vi "Init.vi"(8 "error in (no error)":errorcluster, 11 "Device Descriptor in":string) -> (0 "error out":errorcluster, 3 "PBP Driver":refnum<class "heater_parent.lvclass">)   [LabVIEW 2020, in "Polar Bear Plus All-in-One Plugin.lvlib"]
uses:
  Polar Bear Plus All-in-One Plugin.lvlib
  Typedefs/Init.vi States.ctl
  <instrlib>/RxnRover/Driver Polar Bear Plus/heater_flow_synthesiser/heater_flow_synthesiser.lvclass
  <instrlib>/RxnRover/Driver Polar Bear Plus/heater_explorer/heater_explorer.lvclass
  <instrlib>/RxnRover/Driver Polar Bear Plus/heater_parent/heater_parent.lvclass
  C:/Program Files (x86)/National Instruments/LabVIEW 2020/instr.lib/RxnRover/Driver Polar Bear Plus/heater_parent/heater_parent.lvclass
panel:
  in  "Device Type":string(combo)="PBP Flow Synthesiser"
  in  "IP Address":string
  in  "Connect Btn":bool
  # "1. Device Type"
  # "2. Device IP Address"
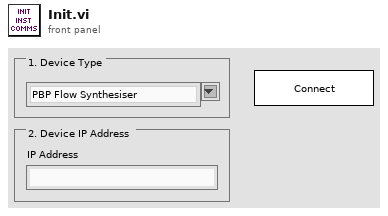
[diagram p1: front panel]
types:
  T1 = typedef "Polar Bear Plus All-in-One Plugin.lvlib/Init.vi States.ctl" = enum16{"Waiting for connection", "Connecting", "Successful connection", "Failed to connect", "Closing"}
  T2 = enum32{"Invalid", "Standard", "Closed", "Hidden", "Minimized", "Maximized"}
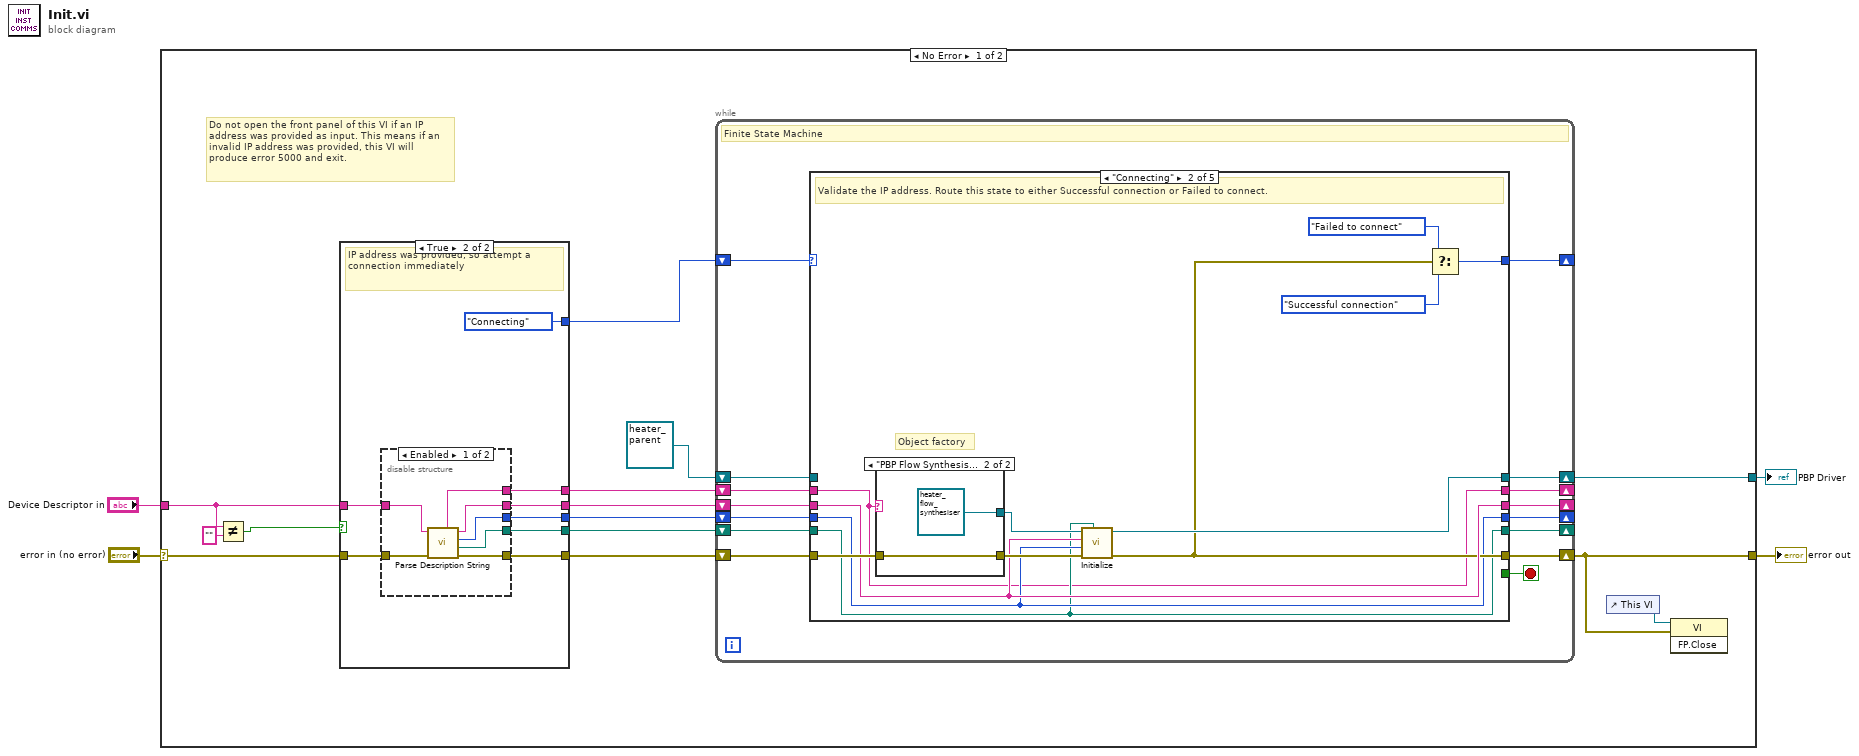
[diagram p0: block diagram]
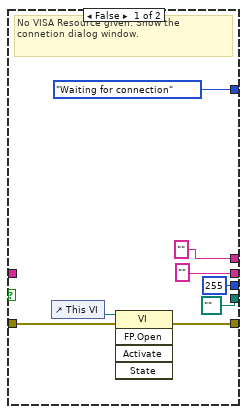
[diagram p2: hidden frame]
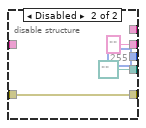
[diagram p3: hidden frame]
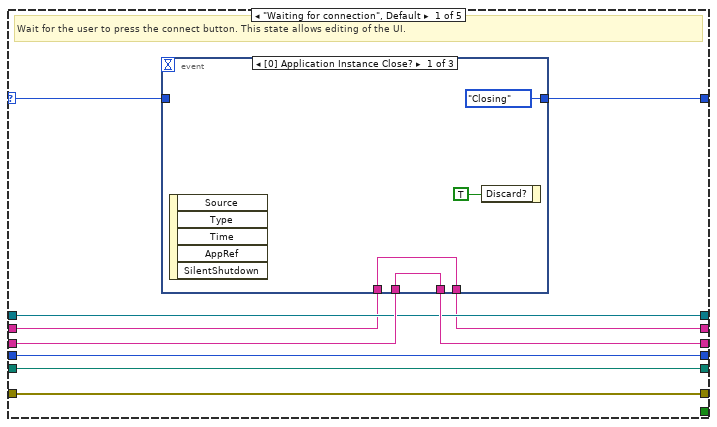
[diagram p4: hidden frame]
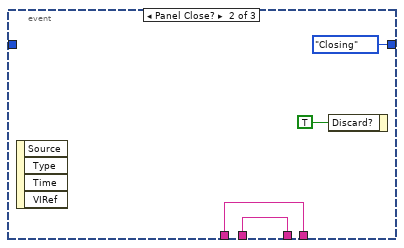
[diagram p5: hidden frame]
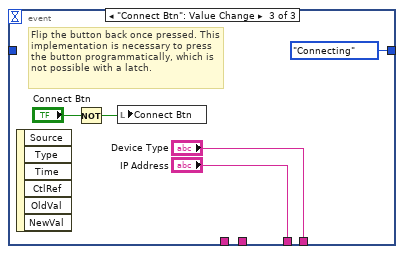
[diagram p6: hidden frame]
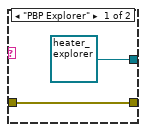
[diagram p7: hidden frame]
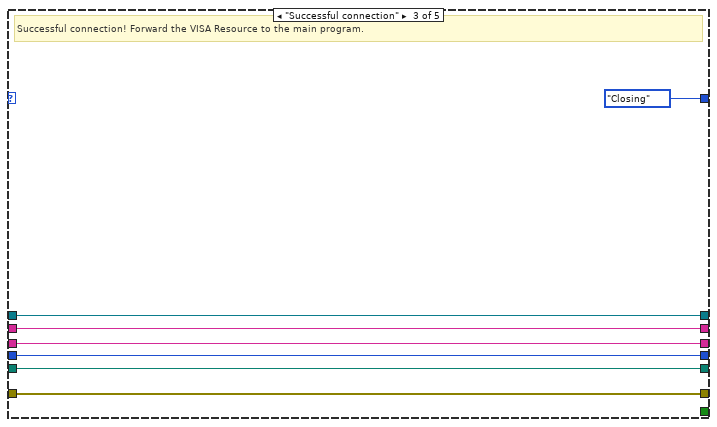
[diagram p8: hidden frame]
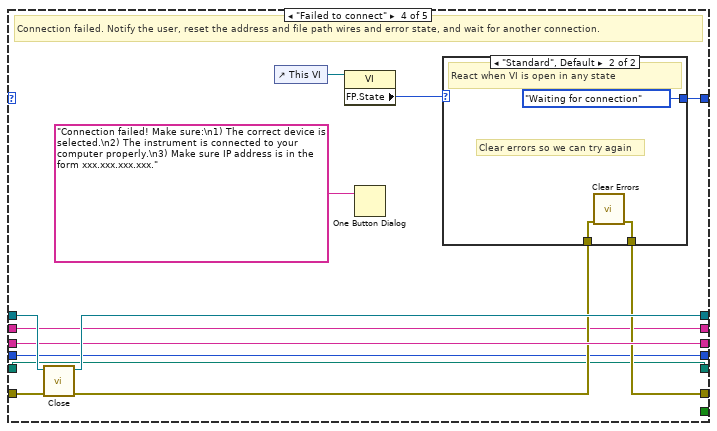
[diagram p9: hidden frame]
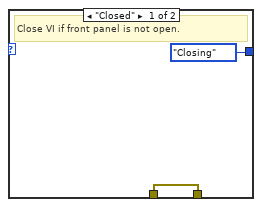
[diagram p10: hidden frame]
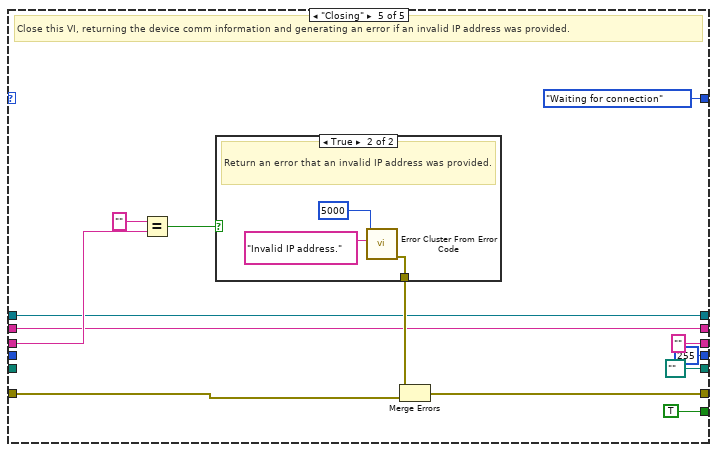
[diagram p11: hidden frame]
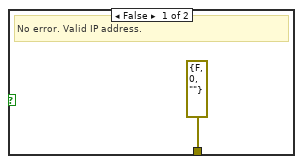
[diagram p12: hidden frame]
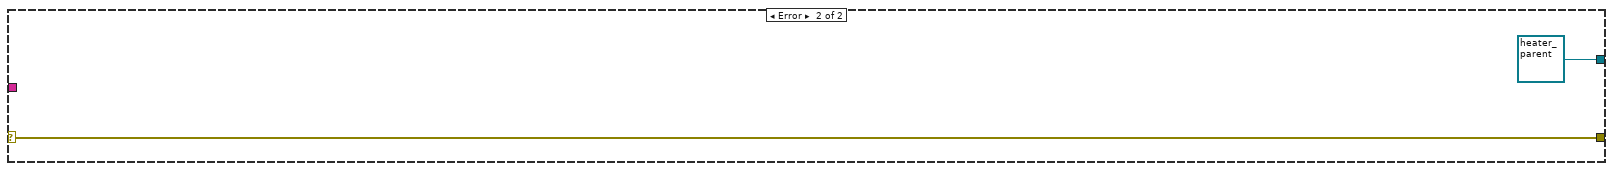
[diagram p13: hidden frame]
diagram:
  n1 = case shown="No Error" "error in (no error)" {
    selector: "error in (no error)" -> [w15 w143]
    tunnel: [w17 w143] -> w3
    tunnel: "Device Descriptor in" -> [w12 _]
    tunnel: [w10 refnum<class "heater_parent.lvclass"> refnum ("polar_bear_plus_drivers.lvlib:heater_parent.lvclass")] -> w1
    frame No Error {
      # "Do not open the front panel of this VI if an IP address was provided as input. This means if an invalid IP address was provided, this VI will produce error 5000 and exit."
      n2 = Not Equal?(x=w12, y="" ("x")) -> (x != y?=w9:bool)
      n3 = case shown="True" w9 {
        tunnel: w15 -> [w25 w34]
        tunnel: [w24 w32] -> w14
        tunnel: [Init.vi_States."Waiting for connection" Init.vi_States."Connecting"] -> w13
        tunnel: w12 -> [_ w31]
        tunnel: ["" ("READ;WRITE Files in") w30] -> w11
        tunnel: [u8 255 ("Modbus Address") w29] -> w7
        tunnel: [path "" ("Data Directory") w28] -> w6
        tunnel: ["" ("READ;WRITE Files in") w27] -> w5
        frame False {
          # "No VISA Resource given. Show the connetion dialog window."
          n4 = control-ref of="This VI"() -> (w26:refnum<vi>)
          n5 = invoke class="VI" method="FP.Open"(reference=w26, error in=w25) -> (error out=w24:errorcluster)  [unwired: 3 in, 4 out]
        }
        frame True {
          # "IP address was provided, so attempt a connection immediately"
          n6 = disable-structure shown="Enabled" {
            disable-tunnel: w34 -> [w41 w42]
            disable-tunnel: [w40 w42] -> w32
            disable-tunnel: w31 -> [w39 _]
            disable-tunnel: [w38 "" ("IP Address")] -> w30
            disable-tunnel: [w37 u8 255 ("Modbus Address")] -> w29
            disable-tunnel: [w36 path "" ("Data Directory")] -> w28
            disable-tunnel: [w35 _] -> w27
            frame Enabled {
              n7 = call <instrlib>:"Parse Description String.vi"("error in (no error)"=w41, "Description String"=w39) -> ("error out"=w40:errorcluster, "Data Directory"=w36:path, "Modbus Address"=w37:u8, "IP Address"=w38:string, "Device Type"=w35:string)  [unwired: 5 in]
            }
            frame Disabled {
            }
          }
        }
      }
      n8 = while {
        shift-right: [w59] -> _
        shift-left: w13 -> [w60]
        shift-right: [w52] -> _
        shift-left: w11 -> [w57]
        shift-right: [w55] -> w17
        shift-left: w14 -> [w56]
        shift-right: [w54] -> w10
        shift-left: refnum<class "heater_parent.lvclass"> refnum ("polar_bear_plus_drivers.lvlib:heater_parent.lvclass") -> [w53]
        shift-right: [w49] -> _
        shift-left: w7 -> [w51]
        shift-right: [w48] -> _
        shift-left: w6 -> [w50]
        shift-right: [w47] -> _
        shift-left: w5 -> [w46]
        stop <- w58 stop-if-true
        # "Finite State Machine"
        n9 = case shown="\"Connecting\"" w60 {
          selector: w60 -> [w70 _ _ _ _]
          tunnel: [w69 w95 Init.vi_States."Closing" w119 Init.vi_States."Waiting for connection"] -> w59
          tunnel: [_ _ _ _ TRUE] -> w58
          tunnel: [w65 w89 w104 w113 w131] -> w54
          tunnel: w57 -> [w67 w88 w103 w112 w135]
          tunnel: w56 -> [w68 w92 w105 w115 w132]
          tunnel: [w68 w87 w105 w110 w133] -> w55
          tunnel: w53 -> [w65 _ w104 w114 w131]
          tunnel: [w66 w88 w103 w112 "" ("READ;WRITE Files in")] -> w52
          tunnel: w51 -> [w64 w86 w102 w109 _]
          tunnel: w50 -> [w63 w85 w101 w108 _]
          tunnel: [w64 w86 w102 w109 u8 255 ("Modbus Address")] -> w49
          tunnel: [w63 w85 w101 w108 path "" ("Data Directory")] -> w48
          tunnel: [w62 w84 w100 w107 w125] -> w47
          tunnel: w46 -> [w61 w84 w100 w107 w125]
          frame "Waiting for connection", Default {
            # "Wait for the user to press the connect button. This state allows editing of the UI."
            n10 = event shown="[0] Application Instance Close?" {
              selector: _ -> [_ _ _]
              dyn-events: _ -> [_ _ _]
              timeout: _ -> [_ _ _]
              tunnel: [Init.vi_States."Closing" Init.vi_States."Closing" Init.vi_States."Connecting"] -> w69
              tunnel: w70 -> [_ _ _]
              tunnel: w67 -> [w72 w76 _]
              tunnel: [w72 w76 "IP Address"] -> w66
              tunnel: [w71 w75 "Device Type"] -> w62
              tunnel: w61 -> [w71 w75 _]
              event Application Instance Close? {
                n11 = event-data() -> ()  [unwired: 1 in, 5 out]
                n12 = event-data("Discard?"=TRUE) -> ()  [unwired: 1 in, 1 out]
              }
              event Panel Close? {
                n13 = event-data() -> ()  [unwired: 1 in, 4 out]
                n14 = event-data("Discard?"=TRUE) -> ()  [unwired: 1 in, 1 out]
              }
              event "Connect Btn": Value Change {
                # "Flip the button back once pressed. This implementation is necessary to press the button programmatically, which is not possible with a latch."
                n15 = event-data() -> ()  [unwired: 1 in, 6 out]
                n16 = Not(x="Connect Btn") -> (.not. x?=w81:bool)
                n17 = local write "Connect Btn"(w81) -> ()
              }
            }
          }
          frame "Connecting" {
            # "Object factory"
            # "Validate the IP address. Route this state to either Successful connection or Failed to connect."
            n18 = case shown="\"PBP Flow Synthesiser\", Default" w84 {
              tunnel: w92 -> [w97 w99]
              tunnel: [w97 w99] -> w91
              tunnel: [refnum<class "heater_explorer.lvclass"> refnum ("polar_bear_plus_drivers.lvlib:heater_explorer.lvclass") refnum<class "heater_flow_synthesiser.lvclass"> refnum ("polar_bear_plus_drivers.lvlib:heater_flow_synthesiser.lvclass")] -> w90
              frame "PBP Explorer" {
              }
              frame "PBP Flow Synthesiser", Default {
              }
            }
            n19 = call-dynamic "Initialize.vi"("start path"=w85, "error in (no error)"=w91, "Modbus Address"=w86, "IP Address"=w88, "vici_flow_actuator_parent in"=w90) -> ("error out"=w87:errorcluster, "vici_flow_actuator_parent out"=w89:refnum<class "heater_parent.lvclass">)  [unwired: 4 in, 1 out]
            n20 = Select(t=Init.vi_States."Failed to connect", s=w87, f=Init.vi_States."Successful connection") -> (s? t:f=w95:T1)
          }
          frame "Successful connection" {
            # "Successful connection! Forward the VISA Resource to the main program."
          }
          frame "Failed to connect" {
            # "Connection failed. Notify the user, reset the address and file path wires and error state, and wait for another connection."
            n21 = call-dynamic "Close.vi"("error in (no error)"=w115, "heater_parent in"=w114) -> ("error out"=w111:errorcluster, "heater_parent out"=w113:refnum<class "heater_parent.lvclass">)  [unwired: 8 in]
            n22 = control-ref of="This VI"() -> (w117:refnum<vi>)
            n23 = property class="VI"(reference=w117) -> ("FP.State"=w116:T2)  [unwired: 1 in, 2 out]
            n24 = One Button Dialog(message="Connection failed! Make sure:\n1) The correct device is selected.\n2) The instrument is connected to your computer properly.\n3) Make sure IP address is in the form xxx.xxx.xxx.xxx.") -> ()  [unwired: 1 in, 1 out]
            n25 = case shown="\"Standard\", Default" w116 {
              tunnel: [Init.vi_States."Closing" Init.vi_States."Waiting for connection"] -> w119
              tunnel: w111 -> [w120 w123]
              tunnel: [w120 w122] -> w110
              frame "Closed" {
                # "Close VI if front panel is not open."
              }
              frame "Standard", Default {
                # "Clear errors so we can try again"
                # "React when VI is open in any state"
                n26 = call <vilib>:"Clear Errors.vi"("error in (no error)"=w123) -> ("error out"=w122:errorcluster)  [unwired: 5 in, 1 out]
              }
            }
          }
          frame "Closing" {
            # "Close this VI, returning the device comm information and generating an error if an invalid IP address was provided."
            n27 = Equal?(x="" ("VISA resource in"), y=w135) -> (x = y?=w128:bool)
            n28 = case shown="True" w128 {
              tunnel: [errorcluster {"status"=FALSE, "code"=0, "source"=""} ("error out") w140] -> w134
              frame False {
                # "No error. Valid IP address."
              }
              frame True {
                # "Return an error that an invalid IP address was provided."
                n29 = call <vilib>:"Error Cluster From Error Code.vi"("error message (\"\")"="Invalid IP address." ("error message (\"\")"), "error code (0)"=5000) -> ("error out"=w140:errorcluster)  [unwired: 7 in]
              }
            }
            n30 = Merge Errors(w134, w132) -> (w133:errorcluster)
          }
        }
      }
      n31 = control-ref of="This VI"() -> (w18:refnum<vi>)
      n32 = invoke class="VI" method="FP.Close"(reference=w18, error in=w17) -> ()  [unwired: 1 in, 3 out]
    }
    frame Error {
    }
  }
  "error out" <- w3
  "PBP Driver" <- w1
